vi "howtotruncateanarray.vi"() -> ()   [LabVIEW 2013]
panel:
  in  "Boolean":bool
  out "Histogram 3":u32[](graph)
  out "Histogram 2":u32[](graph)
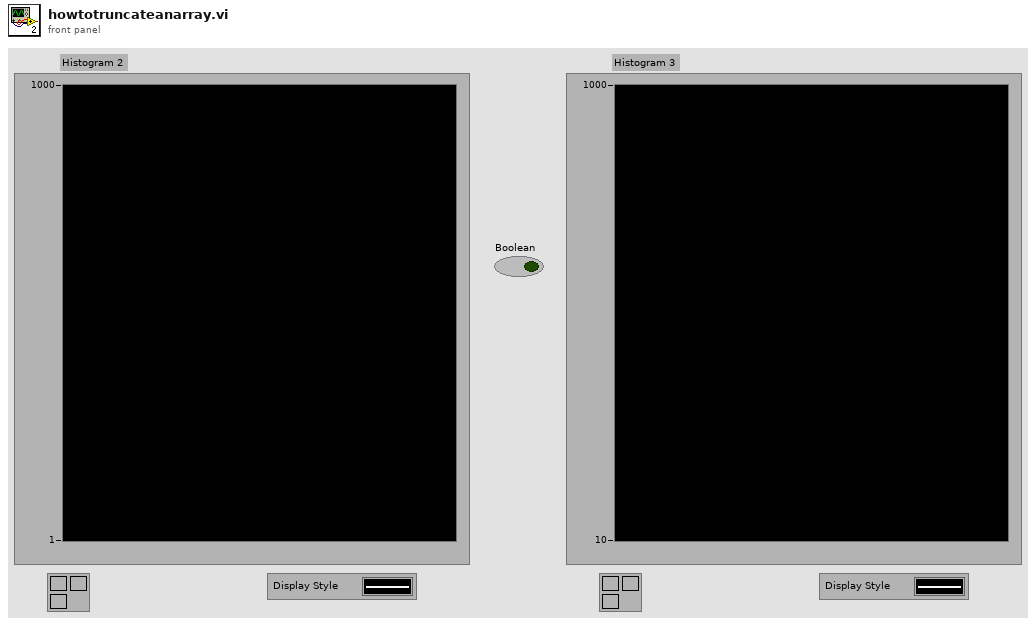
[diagram p1: front panel]
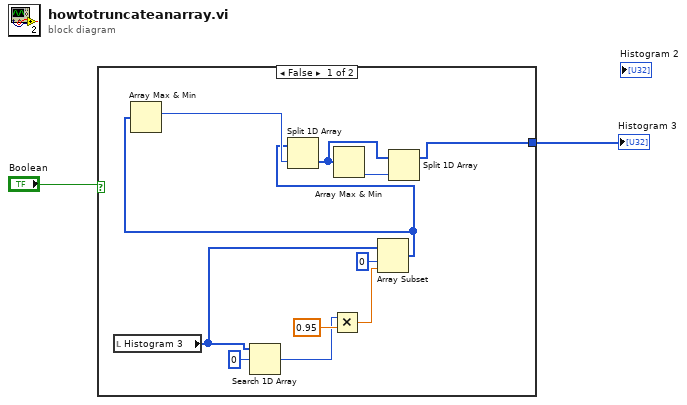
[diagram p0: block diagram]
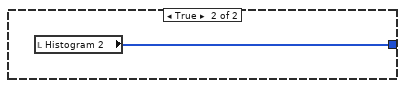
[diagram p2: hidden frame]
diagram:
  n1 = case shown="False" "Boolean" {
    tunnel: [w10 w14] -> w2
    frame False {
      n2 = local read "Histogram 3"() -> (w3:u32[])
      n3 = Search 1D Array(1D array=w3, element=u32 0) -> (index of element=w4:i32)  [unwired: 1 in]
      n4 = Multiply(x=w4, y=0.95) -> (x*y=w9:dbl)
      n5 = Array Subset(array=w3, index=0, length=w9) -> (w6:u32[])
      n6 = Array Max & Min(array=w6) -> (max index (indices)=w13:i32)  [unwired: 3 out]
      n7 = Split 1D Array(array=w6, index=w13) -> (second subarray=w11:u32[])  [unwired: 1 out]
      n8 = Array Max & Min(array=w11) -> (min index (indices)=w12:i32)  [unwired: 3 out]
      n9 = Split 1D Array(array=w11, index=w12) -> (first subarray=w10:u32[])  [unwired: 1 out]
    }
    frame True {
      n10 = local read "Histogram 2"() -> (w14:u32[])
    }
  }
  "Histogram 3" <- w2
